vi "Handle Error.vi"(8 "error in (no error)":errorcluster, 11 "Measure Object in":refnum<class "Template Module.lvclass">) -> (0 "error out":errorcluster, 2 "stop actor?":bool=TRUE, 3 "Measure Object out":refnum<class "Template Module.lvclass">)   [LabVIEW 2020, in "Template Module.lvclass"]
doc: "(<B>Filename</B>: Actor Framework.lvlib:Actor.lvclass:Handle Error.vi)\n\nDefines how the actor handles an error that occurred while processing a message. By default, this method does nothing except stop the actor."
uses:
  Template Module.lvclass
  C:/Program Files/National Instruments/LabVIEW 2020/vi.lib/ActorFramework/Actor/Actor.lvclass
  <vilib>/ActorFramework/Actor/Actor.lvclass/Actor.ctl
  <vilib>/ActorFramework/Report Error Msg/Report Error Msg.lvclass/Report Error Msg.ctl
  <vilib>/ActorFramework/Message Enqueuer/Message Enqueuer.lvclass/Message Enqueuer.ctl
  <vilib>/ActorFramework/Message Enqueuer/Enqueue.vi
  <vilib>/ActorFramework/Report Error Msg/Report Error Msg.lvclass
  C:/Program Files/National Instruments/LabVIEW 2020/vi.lib/ActorFramework/Message/Message.lvclass
  <vilib>/ActorFramework/Message Priority Queue/Priority Enqueue.vi
  <vilib>/ActorFramework/Message Enqueuer/Message Enqueuer.lvclass
  Template Module.lvclass/Template Module.ctl
  <vilib>/ActorFramework/Actor/Actor.lvclass
  Controllers/Application Controller Messages/Display Error Msg/Display Error Msg.lvclass
  C:/GitHub/LabActor/Template Module/Template Module.lvclass
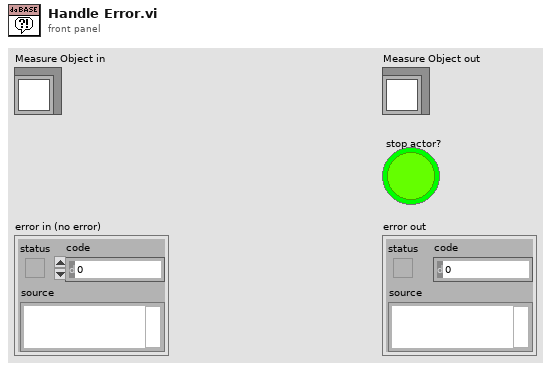
[diagram p1: front panel]
types:
  T1 = typedef "LabActor Error.ctl" = cluster{"Time":string, "Message":string, "Source":string, "Code":i32, "Error?":bool, "Module":string, "Formated Message":string}
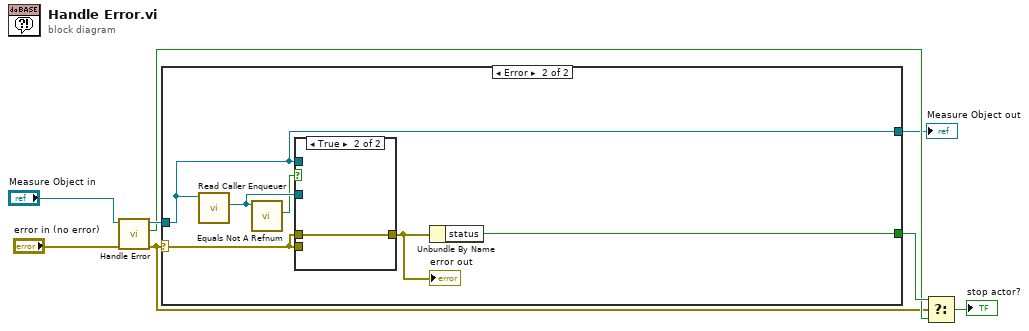
[diagram p0: block diagram]
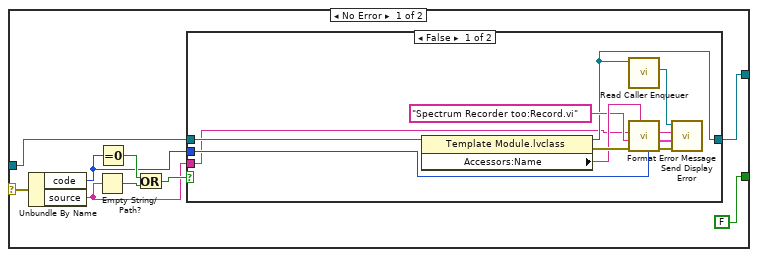
[diagram p2: hidden frame]
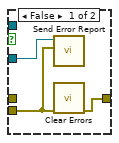
[diagram p4: hidden frame]
diagram:
  n1 = call-parent "Handle Error.vi"("error in (no error)"="error in (no error)", "Actor in"="Measure Object in") -> ("error out"=w1:errorcluster, "stop actor?"=w4:bool, "Actor out"=w6:refnum<class "Template Module.lvclass">)  [unwired: 7 in]
  n2 = case shown="Error" w1 {
    selector: w1 -> [w16 w32]
    tunnel: w6 -> [w12 w33]
    tunnel: [FALSE w30] -> w5
    tunnel: [w11 w33] -> w2
    frame No Error {
      n3 = Unbundle By Name(w16) -> ("code"=w9:i32, "source"=w10:string)
      n4 = Empty String/Path?(string/path=w10) -> (empty?=w13:bool)
      n5 = Equal To 0?(x=w9) -> (x = 0?=w14:bool)
      n6 = Or(x=w14, y=w13) -> (x .or. y?=w15:bool)
      n7 = case shown="False" w15 {
        tunnel: w12 -> [w21 w29]
        tunnel: [w20 w29] -> w11
        tunnel: w10 -> [w18 _]
        tunnel: w9 -> [w19 _]
        frame False {
          n8 = property class="Template Module.lvclass"(reference=w21) -> (reference out=w20:refnum<class "Template Module.lvclass">, error out=w26:errorcluster, "Accessors:Name"=w24:string)  [unwired: 1 in]
          n9 = call <vilib>:"Read Caller Enqueuer.vi"("Actor"=w20) -> ("Caller Enqueuer"=w23:refnum<class "Message Enqueuer.lvclass">)  [unwired: 10 in]
          n10 = call "Format Error Message.vi"("Code"=w19, "Module"=w24, "error in"=w26, "Source"="Spectrum Recorder too:Record.vi", "Message"=w18) -> ("error out"=w27:errorcluster, "LabActor Error"=w28:T1, "Formated error message"=w25:string)  [unwired: 4 in]
          n11 = call "Send Display Error.vi"("error in (no error)"=w27, "LabActor Error"=w28, "Error message"=w25, "Message Enqueuer"=w23) -> ()  [unwired: 6 in, 2 out]
        }
        frame True {
        }
      }
    }
    frame Error {
      n12 = call <vilib>:"Read Caller Enqueuer.vi"("Actor"=w33) -> ("Caller Enqueuer"=w35:refnum<class "Message Enqueuer.lvclass">)  [unwired: 10 in]
      n13 = call <vilib>:"Equals Not A Refnum.vi"("Message Enqueuer"=w35) -> ("Not a refnum?"=w34:bool)  [unwired: 10 in]
      n14 = case shown="True" w34 {
        tunnel: w32 -> [_ w39]
        tunnel: [w38 w39] -> w31
        tunnel: w35 -> [w37 _]
        tunnel: w33 -> [_ _]
        tunnel: w32 -> [w36 _]
        frame False {
          n15 = call <vilib>:"Send Error Report.vi"("Error From Sender"=w36, "Message Enqueuer"=w37) -> ()  [unwired: 9 in, 1 out]
          n16 = call <vilib>:"Clear Errors.vi"("error in (no error)"=w36) -> ("error out"=w38:errorcluster)  [unwired: 5 in, 1 out]
        }
        frame True {
        }
      }
      "error out" <- w31
      n17 = Unbundle By Name(w31) -> ("status"=w30:bool)
    }
  }
  "Measure Object out" <- w2
  n18 = Select(t=w5, s=w1, f=w4) -> (s? t:f=→"stop actor?":bool)
